vi "Averaged Cross Spectrum (Real-Im).vi"(0 "scaled signal X [EUx]":dbl[](array[numeric]) format="%.2f", 1 "window":T6=1 items=["None"=0, "Hanning"=1, "Hamming"=2, "Blackman-Harris"=3, "Exact Blackman"=4, "Blackman"=5, "Flat Top"=6, "4 Term B-Harris "=7, "7 Term B-Harris"=8, "Low Sidelobe"=9, "Force - Exponential"=10, "Blackman Nuttall"=11, "Triangle"=30, "Bartlett-Hanning"=31, "Bohman"=32, "Parzen"=33, "Welch"=34, "Kaiser"=60, "Dolph-Chebyshev"=61, "Gaussian"=62], 2 "force/exp settings":T5={"force window [%]"=50.0, "exponential window [%]"=10.0} {"exponential window [%]" min=0.0 max=100.0 format="%.2f"; "force window [%]" min=0.0 max=100.0 format="%.2f"}, 5 "scaled signal Y [EUy]":dbl[](array[numeric]) format="%.2f", 7 "sampling frequency [Hz]":dbl=10000.0 format="%.2f", 9 "channel X info":T2={"sensor sensitivity [mV/EU]"=1000.0, "engineering units"=1, "dB reference [EU]"=1.0, "custom label"="EU", "weighting filter"=0, "pregain [dB]"=0.0} {"pregain [dB]" format="%.2f"; "weighting filter" items=["Linear", "A-weighting", "B-weighting", "C-weighting", "ITU-R 468-4", "Dolby", "CCITT", "C-message"]; "dB reference [EU]" format="%^.1e"; "engineering units" items=["custom..."=0, "V"=1, "A"=21, "Pa"=2, "N"=20, "g"=3, "m/s^2"=4, "m/s"=5, "m"=6, "mm/s"=12, "mm"=13, "microns/s"=14, "microns"=15, "in/s^2"=7, "in/s"=8, "in"=9, "mils/s"=10, "mils"=11, "rad/s^2"=16, "rad/s"=17, "rad"=18, "strain"=19]; "sensor sensitivity [mV/EU]" format="%.2f"}, 11 "channel Y info":T2={"sensor sensitivity [mV/EU]"=1000.0, "engineering units"=1, "dB reference [EU]"=1.0, "custom label"="EU", "weighting filter"=0, "pregain [dB]"=0.0} {"pregain [dB]" format="%.2f"; "weighting filter" items=["Linear", "A-weighting", "B-weighting", "C-weighting", "ITU-R 468-4", "Dolby", "CCITT", "C-message"]; "dB reference [EU]" format="%^.1e"; "engineering units" items=["custom..."=0, "V"=1, "A"=21, "Pa"=2, "N"=20, "g"=3, "m/s^2"=4, "m/s"=5, "m"=6, "mm/s"=12, "mm"=13, "microns/s"=14, "microns"=15, "in/s^2"=7, "in/s"=8, "in"=9, "mils/s"=10, "mils"=11, "rad/s^2"=16, "rad/s"=17, "rad"=18, "strain"=19]; "sensor sensitivity [mV/EU]" format="%.2f"}, 12 "reset averaging (T)":bool=TRUE, 13 "averaging parameters":T1={"averaging mode"=enum."RMS averaging", "weighting mode"=enum."Linear", "number of averages"=10} {"number of averages" min=1}) -> (3 "df [Hz]":dbl format="%.2f", 4 "real part [EUx EUy rms]":dbl[](array[numeric]) format="%.2f", 6 "imaginary part [EUx EUy rms]":dbl[](array[numeric]) format="%.2f", 8 "unit label":string, 10 "averages completed":dbl format="%.2f", 14 "window constants":cluster{"eq noise BW":dbl, "coherent gain":dbl} {"coherent gain" format="%.2f"; "eq noise BW" format="%.2f"}, 15 "error out":errorcluster)   [LabVIEW 2017]
doc: "Computes the averaged cross power spectrum of the input signals. Typically, X signal is the stimulus, and Y signal is the response of the system. Results are returned as real and imaginary parts.\nEach block of data corresponds to a single FFT block and has to be passed individually to this VI. The first time this VI is called, reset averaging must be TRUE (default value), to start a new averaging process. For subsequent calls, reset averaging must be FALSE to continue the averaging process. Averages completed returns the number of averages completed so far.\nAveraging parameters specifies how the averaging is performed. This includes the averaging mode (no averaging, vector averaging or RMS averaging), the weighting mode (linear or exponential) and the number of averages (used only if the weighting mode is exponential)."
uses:
  <vilib>/addons/_NISVFA/_Shared subVIs/Controls/svc_Window [Dual FFT].ctl
  <vilib>/addons/Sound and Vibration/compatibility/Controls/svl_Channel Info.ctl
  <vilib>/addons/Sound and Vibration/compatibility/Controls/svl_Engineering Units Text Ring.ctl
  <vilib>/addons/Sound and Vibration/compatibility/Controls/svl_Weighting Filter Text Ring.ctl
  <vilib>/Analysis/4window.llb/Force Window (DBL).vi
  <vilib>/Analysis/4window.llb/Exponential Window (DBL).vi
  <vilib>/Analysis/2dsp.llb/Cross Power (DBL).vi
  <vilib>/Analysis/2dsp.llb/Real FFT.vi
  <vilib>/Analysis/0measdsp.llb/Scaled Time Domain Window (DBL).vi
  <vilib>/Analysis/NI_AALPro.lvlib
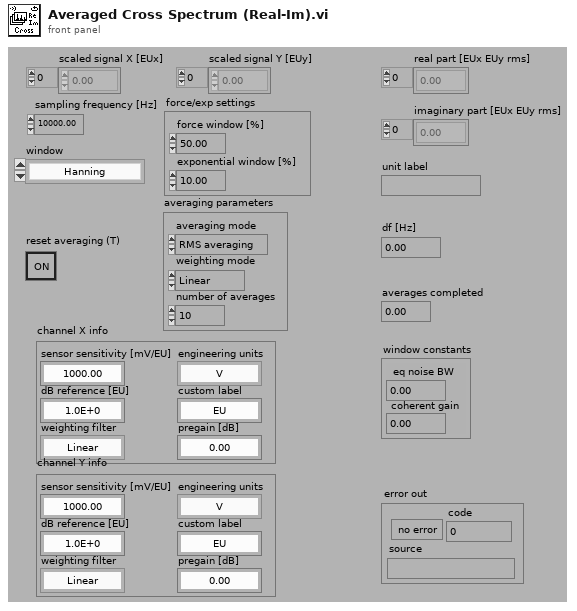
[diagram p1: front panel]
types:
  T1 = cluster{"averaging mode":enum16{"No averaging", "Vector averaging", "RMS averaging"}, "weighting mode":enum16{"Linear", "Exponential"}, "number of averages":u32}
  T2 = typedef "svl_Channel Info.ctl" = cluster{"sensor sensitivity [mV/EU]":dbl, "engineering units":T3, "dB reference [EU]":dbl, "custom label":string, "weighting filter":T4, "pregain [dB]":dbl}
  T3 = typedef "svl_Engineering Units Text Ring.ctl" = u16
  T4 = typedef "svl_Weighting Filter Text Ring.ctl" = u16
  T5 = cluster{"force window [%]":dbl, "exponential window [%]":dbl}
  T6 = typedef "svc_Window [Dual FFT].ctl" = u32
  T7 = enum16{"No averaging", "Vector averaging", "RMS averaging"}
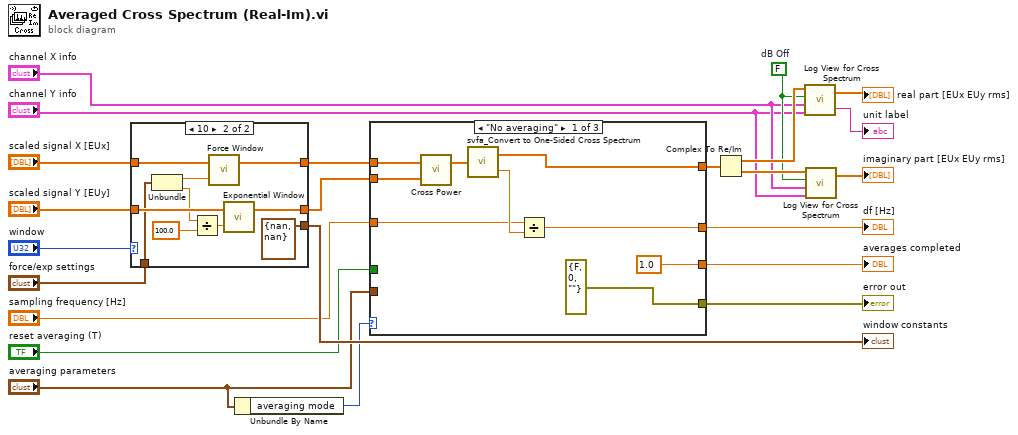
[diagram p0: block diagram]
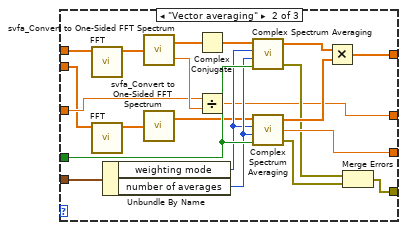
[diagram p2: hidden frame]
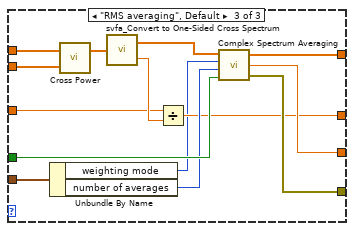
[diagram p3: hidden frame]
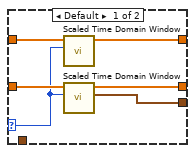
[diagram p4: hidden frame]
diagram:
  w16 = FALSE  # dB Off
  n1 = case shown="10" "window" {
    selector: "window" -> [w24 _]
    tunnel: "scaled signal X [EUx]" -> [w29 w39]
    tunnel: "scaled signal Y [EUy]" -> [w28 w38]
    tunnel: "force/exp settings" -> [_ w34]
    tunnel: [w27 w36] -> w5
    tunnel: [w26 w35] -> w6
    tunnel: [w25 cluster{"eq noise BW":dbl, "coherent gain":dbl} {"eq noise BW"=nan, "coherent gain"=nan} ("window constants")] -> w13
    frame Default {
      n2 = call-poly <vilib>:"Scaled Time Domain Window.vi"("window"=w24, "X"=w29) -> ("Windowed X"=w27:dbl[])  [unwired: 7 in, 2 out]
      n3 = call-poly <vilib>:"Scaled Time Domain Window.vi"("window"=w24, "X"=w28) -> ("window properties"=w25:cluster{"eq noise BW":dbl, "coherent gain":dbl}, "Windowed X"=w26:dbl[])  [unwired: 7 in, 1 out]
    }
    frame 10 {
      n4 = Unbundle(w34) -> ("force window [%]"=w33:dbl, "exponential window [%]"=w32:dbl)
      n5 = Divide(x=w32, y=100.0 ("x")) -> (x/y=w37:dbl)
      n6 = call-poly <vilib>:"Force Window.vi"("duty cycle(%)"=w33, "X"=w39) -> ("Windowed X"=w36:dbl[])  [unwired: 1 out]
      n7 = call-poly <vilib>:"Exponential Window.vi"("final value"=w37, "X"=w38) -> ("Windowed X"=w35:dbl[])  [unwired: 1 out]
    }
  }
  "window constants" <- w13
  n8 = Unbundle By Name("averaging parameters") -> ("averaging mode"=w10:T7)
  n9 = case shown="\"No averaging\"" w10 {
    tunnel: w5 -> [w44 w55 w75]
    tunnel: w6 -> [w43 w51 w74]
    tunnel: "sampling frequency [Hz]" -> [w42 w53 w73]
    tunnel: [w40 w52 w71] -> w3
    tunnel: [w41 w63 w80] -> w4
    tunnel: "reset averaging (T)" -> [_ w67 w83]
    tunnel: "averaging parameters" -> [_ w68 w82]
    tunnel: [1.0 ("averages completed") w65 w79] -> w2
    tunnel: [errorcluster {"status"=FALSE, "code"=0, "source"=""} ("error out") w61 w78] -> w1
    frame "No averaging" {
      n10 = call-poly <vilib>:"Cross Power.vi"("Y"=w43, "X"=w44) -> ("Sxy"=w45:cdb[])  [unwired: 1 out]
      n11 = call <vilib>:"svfa_Convert to One-Sided Cross Spectrum.vi"("two-sided cross spectrum"=w45) -> ("one-sided cross spectrum"=w41:cdb[], "block size"=w46:dbl)
      n12 = Divide(x=w42, y=w46) -> (x/y=w40:dbl)
    }
    frame "Vector averaging" {
      n13 = call-poly <vilib>:"FFT.vi"("X"=w55) -> ("FFT {X}"=w57:cdb[])  [unwired: 9 in, 1 out]
      n14 = call-poly <vilib>:"FFT.vi"("X"=w51) -> ("FFT {X}"=w50:cdb[])  [unwired: 9 in, 1 out]
      n15 = Unbundle By Name(w68) -> ("weighting mode"=w60:enum16{"Linear", "Exponential"}, "number of averages"=w66:u32)
      n16 = call <vilib>:"svfa_Convert to One-Sided FFT Spectrum.vi"("two-sided FFT spectrum"=w57) -> ("one-sided FFT spectrum"=w54:cdb[], "block size"=w56:dbl)
      n17 = call <vilib>:"svfa_Convert to One-Sided FFT Spectrum.vi"("two-sided FFT spectrum"=w50) -> ("one-sided FFT spectrum"=w49:cdb[])  [unwired: 1 out]
      n18 = Complex Conjugate(1:w54) -> (0:w69:cdb[])
      n19 = Divide(x=w53, y=w56) -> (x/y=w52:dbl)
      n20 = call <vilib>:"Complex Spectrum Averaging.vi"("reset averaging (T)"=w67, "number of averages"=w66, "weighting mode"=w60, "complex spectrum"=w69) -> ("error out"=w59:errorcluster, "averaged complex spectrum"=w64:cdb[])  [unwired: 1 out]
      n21 = call <vilib>:"Complex Spectrum Averaging.vi"("reset averaging (T)"=w67, "number of averages"=w66, "weighting mode"=w60, "complex spectrum"=w49) -> ("error out"=w58:errorcluster, "averages completed"=w65:dbl, "averaged complex spectrum"=w62:cdb[])
      n22 = Multiply(x=w64, y=w62) -> (x*y=w63:cdb[])
      n23 = Merge Errors(w59, w58) -> (w61:errorcluster)
    }
    frame "RMS averaging", Default {
      n24 = Unbundle By Name(w82) -> ("weighting mode"=w70:enum16{"Linear", "Exponential"}, "number of averages"=w81:u32)
      n25 = call-poly <vilib>:"Cross Power.vi"("Y"=w74, "X"=w75) -> ("Sxy"=w76:cdb[])  [unwired: 1 out]
      n26 = call <vilib>:"svfa_Convert to One-Sided Cross Spectrum.vi"("two-sided cross spectrum"=w76) -> ("one-sided cross spectrum"=w72:cdb[], "block size"=w77:dbl)
      n27 = Divide(x=w73, y=w77) -> (x/y=w71:dbl)
      n28 = call <vilib>:"Complex Spectrum Averaging.vi"("reset averaging (T)"=w83, "number of averages"=w81, "weighting mode"=w70, "complex spectrum"=w72) -> ("error out"=w78:errorcluster, "averages completed"=w79:dbl, "averaged complex spectrum"=w80:cdb[])
    }
  }
  "df [Hz]" <- w3
  "averages completed" <- w2
  "error out" <- w1
  n29 = Complex To Re/Im(x + iy=w4) -> (x=w19:dbl[], y=w18:dbl[])
  n30 = call <vilib>:"Log View for Cross Spectrum.vi"("channel Y info"="channel Y info", "channel X info"="channel X info", "dB On (T)"=w16, "cross spectrum [EUx EUy rms]"=w19) -> ("unit label"=→"unit label":string, "log view cross spectrum [dB EUx EUy]"=→"real part [EUx EUy rms]":dbl[])
  n31 = call <vilib>:"Log View for Cross Spectrum.vi"("channel Y info"="channel Y info", "channel X info"="channel X info", "dB On (T)"=w16, "cross spectrum [EUx EUy rms]"=w18) -> ("log view cross spectrum [dB EUx EUy]"=→"imaginary part [EUx EUy rms]":dbl[])  [unwired: 1 out]
